vi "Get Subscribe Data Events.vi"(11 "UserEvents in":refnum<class "UserEvents.lvclass">) -> (2 "Subscribe Data Events":T1, 3 "UserEvents out":refnum<class "UserEvents.lvclass">)   [LabVIEW 2015, in "UserEvents.lvclass"]
uses:
  UserEvents.lvclass
  Typedefs/Subscribe Data Events.ctl
  UserEvents.lvclass/UserEvents.ctl
  Typedefs/FAMT Typedefs.lvlib
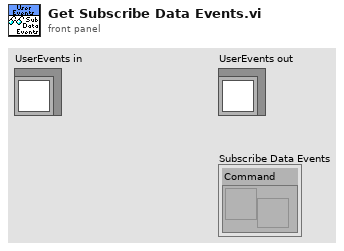
[diagram p1: front panel]
types:
  T1 = typedef "FAMT Typedefs.lvlib/Subscribe Data Events.ctl" = cluster{"Command":refnum<user-event>}
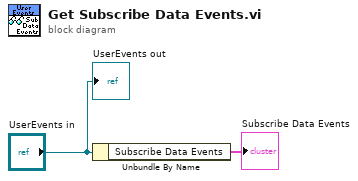
[diagram p0: block diagram]
diagram:
  n1 = Unbundle By Name("UserEvents in") -> ("Subscribe Data Events"=→"Subscribe Data Events":T1)
  "UserEvents out" <- "UserEvents in"
